vi "Vel_Estimate.vi"(9 "gain":dbl=100.0, 10 "Step Size (s)":dbl, 11 "position":dbl) -> (3 "w":dbl)   [LabVIEW 2012]
uses:
  <vilib>/Simulation/Implementation/Shared/SIMSCR Execution Mode.ctl
  <vilib>/Simulation/Scripting/Companion Diagram/SimConfigNode/SimParams.ctl
  <vilib>/Simulation/Scripting/Companion Diagram/SimConfigNode/_simSolvers.ctl
  <vilib>/Simulation/Param Hierarchy/Typedefs/SIMPH Param Control Actions.ctl
  <vilib>/Simulation/Implementation/Shared/NILVSim_ParamChanged.vi
  <vilib>/Simulation/ContinuousLinear/Implementation/NILVSim Transfer Function Direct.llb/SIM Transfer Function Direct (SISO).vi
  <vilib>/Simulation/SignalArithmetic/Implementation/NILVSim Gain.llb/SIM Gain (scalar).vi
  <vilib>/Simulation/DiscreteLinear/Implementation/NILVSim Discrete Integrator Forward.llb/SIM Discrete Integrator Forward Distributor (scalar).vi
  <vilib>/Simulation/Nonlinear/Implementation/NILVSim DeadZone.llb/SIM DeadZone (scalar).vi
  <vilib>/Simulation/DiscreteLinear/Implementation/NILVSim Discrete Integrator Forward.llb/SIM Discrete Integrator Forward Collector (scalar).vi
  <vilib>/Simulation/Implementation/Shared/NILVSim_Manager.vi
  <vilib>/Simulation/Implementation/Shared/NILVSim_FinalizeModel.vi
  <vilib>/Simulation/Implementation/Shared/SIM Unbundle Sim Info.vi
  <vilib>/Utility/error.llb/Clear Errors.vi
  <vilib>/Simulation/Implementation/Shared/NILVSim_GetModelError.vi
  <vilib>/Simulation/Implementation/Shared/SIM SimErrorHandler.vi
  <vilib>/Simulation/Implementation/Shared/SIM Bundle Sim Info.vi
  <vilib>/Simulation/Implementation/Shared/SIMSH Read Queue.vi
  <vilib>/Simulation/Implementation/Shared/NILVSim_Initialize.vi
  <vilib>/Simulation/Utility/Implementation/NILVSim Get Time and IsAcceptedStep.vi
  <vilib>/Simulation/Scripting/Companion Diagram/SimConfigNode/SimDog.xnode
  <vilib>/Simulation/Implementation/XNodeFramework/SimXNode/SimX.xnode
  <vilib>/Simulation/DiscreteLinear/Implementation/NILVSim Discrete Integrator Forward.llb/SIM Discrete Integrator Forward (scalar).vi
  <vilib>/Simulation/Implementation/Shared/NI_SIM_Implementation.lvlib
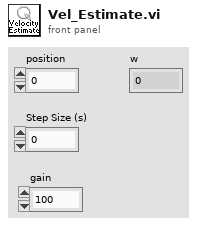
[diagram p1: front panel]
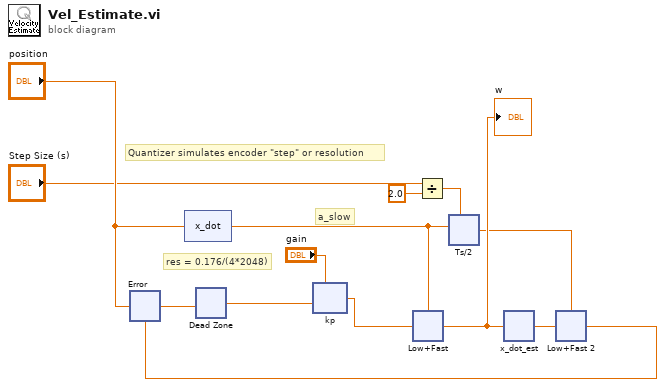
[diagram p0: block diagram]
diagram:
  # "Quantizer simulates encoder \"step\" or resolution"
  # "a_slow"
  # "res = 0.176/(4*2048)"
  n1 = xnode "x_dot"("input u(k)"="position") -> ("output y(k)"=w8:dbl)  [unwired: 4 in, 1 out]
  n2 = Divide ("Divide 2")(x="Step Size (s)", y=2.0 ("y 2")) -> (x/y=w4:dbl)
  n3 = xnode "Ts/2"("gain"=w4, "input"=w8) -> ("output"=w6:dbl)  [unwired: 2 in]
  n4 = xnode "Error"("Operand1"="position", "Operand2"=w9) -> ("Result"=w1:dbl)
  n5 = xnode "Dead Zone"("input"=w1) -> ("output"=w2:dbl)  [unwired: 4 in]
  n6 = xnode "kp"("gain"="gain", "input"=w2) -> ("output"=w10:dbl)  [unwired: 2 in]
  n7 = xnode "Low+Fast"("Operand1"=w8, "Operand2"=w10) -> ("Result"=w12:dbl)
  "w" <- w12
  n8 = xnode "x_dot_est"("input"=w12) -> ("output"=w5:dbl)  [unwired: 10 in, 1 out]
  n9 = xnode "Low+Fast 2"("Operand1"=w6, "Operand2"=w5) -> ("Result"=w9:dbl)
